vi "Objects to table.vi"(8 "error in":errorcluster, 11 "All Objects":set{T1}(c389)) -> (0 "error out":errorcluster, 3 "Table Control":string[][](table))   [LabVIEW 2019]
uses:
  Logger_class/ObjData.ctl
  Logger_class/ObjType.ctl
  Logger_class/Logger.lvclass
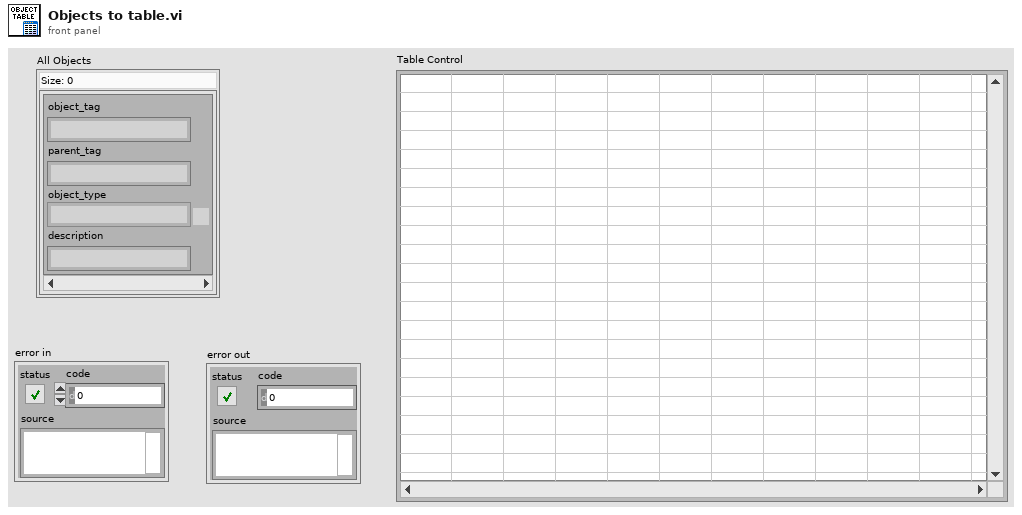
[diagram p1: front panel]
types:
  T1 = typedef "Logger.lvclass/ObjData.ctl" = cluster{"object_tag":string, "parent_tag":string, "object_type":T2, "description":string}
  T2 = typedef "Logger.lvclass/ObjType.ctl" = enum16{"Procces", "Device", "Signal", "DI", "DO", "DA", "AI", "AO", "AA"}
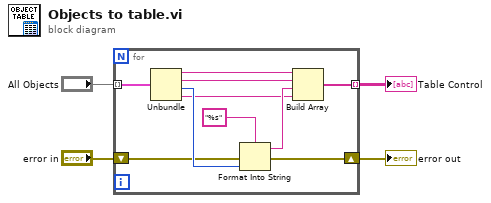
[diagram p0: block diagram]
diagram:
  n1 = for {
    tunnel: "All Objects" -> [w14] mode=indexing
    tunnel: [w7] -> w3 mode=indexing
    shift-right: [w5] -> w1
    shift-left: "error in" -> [w6]
    n2 = Unbundle(w14) -> ("object_tag"=w11:string, "parent_tag"=w10:string, "object_type"=w13:T2, "description"=w8:string)
    n3 = Format Into String(format string="%s", error in=w6, w13) -> (resulting string=w9:string, error out=w5:errorcluster)  [unwired: 1 in]
    n4 = Build Array(w11, w10, w9, w8) -> (w7:string[])
  }
  "Table Control" <- w3
  "error out" <- w1
